vi "Magna Power Constants.vi"() -> ()   [LabVIEW 2012]
panel:
  out "Field Calibration":T1={"Fluke Voltages"=[-0.898, -0.907, -0.921, -0.93, -0.94, -0.952, -0.964, -0.976, -0.988, -1.0, -1.012, -1.025, -1.037, -1.05, -1.062, -1.074, -1.086, -1.099, -1.111, -1.123, -1.135, -1.149, -1.161, -1.174, -1.186, -1.191, -1.197, -1.203, -1.208, -1.214, -1.22, -1.225, -1.23, -1.236, -1.241, -1.246, -1.251, -1.257, -1.263, -1.269, -1.275, -1.28, -1.285, -1.29, -1.295, -1.3, -1.305, -1.309, -1.313, -1.318, -1.322, -1.326, -1.33, -1.334, -1.337, -1.341, -1.344, -1.348, -1.351, -1.354, -1.358, -1.361, -1.364, -1.366, -1.369, -1.372, -1.3748, -1.3775, -1.38, -1.3825, -1.3849, -1.3875, -1.3897, -1.3921, -1.3942, -1.3965, -1.3996, -1.4026, -1.4055, -1.4082, -1.4109, -1.4134, -1.4159, -1.4184, -1.4205, -1.4229, -1.425, -1.4272, -1.4293, -1.4314, -1.4331, -0.9047, -0.9062, -0.913, -0.9163, -0.9235, -0.9271, -0.9341, -0.89598, -0.89247, -0.88898, -0.88568, -0.88203, -0.87833, -0.87495, -0.87474, -0.87134, -0.86785, -0.86466, -0.86127, -0.85792, -0.85453, -0.85123, -0.84792, -0.83742, -0.82773, -0.81808, -0.80865, -0.79937, -0.79043, -0.78145, -0.77261, -0.76419, -0.75595, -0.74795, -0.73984, -0.73183, -0.72447, -0.71682, -0.70957, -0.70236, -0.69555, -0.68879, -0.68235, -0.67601, -0.67006, -0.66447, -0.65904, -0.65409, -0.64949, -0.64665, -0.64399, -0.6411, -0.62648, -0.62463, -0.63583, -0.63404, -0.63113, -0.62861, -0.62767, -0.62314, -0.6205, -0.61798, -0.61351, -0.61151, -0.60949, -0.60732, -0.60535, -0.60349, -0.60167, -0.59983, -0.59814, -0.59651, -0.59498, -0.59348, -0.59204, -0.59063, -0.58928, -0.58803, -0.5868, -0.58563, -0.58455, -0.58349, -0.58248, -0.58145, -0.58051, -0.57962, -0.57872, -0.57781, -0.57701, -0.57621, -0.57545, -0.57468, -0.57434], "Field Values"=[0.00828, 0.0338, 0.0696, 0.1011, 0.1325, 0.1653, 0.1983, 0.2308, 0.2632, 0.297, 0.329, 0.362, 0.394, 0.427, 0.459, 0.489, 0.521, 0.552, 0.584, 0.613, 0.645, 0.678, 0.708, 0.737, 0.767, 0.781, 0.793, 0.808, 0.821, 0.835, 0.849, 0.862, 0.874, 0.887, 0.899, 0.912, 0.923, 0.937, 0.952, 0.966, 0.979, 0.992, 1.004, 1.016, 1.028, 1.039, 1.051, 1.061, 1.072, 1.08, 1.091, 1.1, 1.109, 1.118, 1.127, 1.135, 1.144, 1.152, 1.159, 1.167, 1.175, 1.183, 1.189, 1.197, 1.205, 1.211, 1.218, 1.224, 1.231, 1.236, 1.242, 1.247, 1.253, 1.26, 1.264, 1.27, 1.276, 1.284, 1.29, 1.299, 1.305, 1.311, 1.316, 1.321, 1.327, 1.334, 1.339, 1.343, 1.35, 1.355, 1.361, 0.02542, 0.0298, 0.0499, 0.06, 0.0808, 0.0911, 0.1115, -0.002562, -0.01245, -0.0232, -0.0322, -0.0383, -0.0558, -0.0664, -0.0678, -0.0776, -0.0887, -0.0989, -0.1095, -0.1206, -0.132, -0.1428, -0.1529, -0.1875, -0.2199, -0.2512, -0.285, -0.317, -0.35, -0.38, -0.415, -0.445, -0.477, -0.507, -0.54, -0.573, -0.6, -0.632, -0.662, -0.69, -0.72, -0.749, -0.777, -0.811, -0.838, -0.858, -0.884, -0.908, -0.931, -0.946, -0.958, -0.977, -1.058, -1.068, -1.009, -1.019, -1.024, -1.039, -1.044, -1.074, -1.088, -1.104, -1.123, -1.135, -1.147, -1.159, -1.17, -1.181, -1.192, -1.202, -1.212, -1.222, -1.232, -1.241, -1.249, -1.258, -1.266, -1.274, -1.282, -1.289, -1.296, -1.303, -1.309, -1.314, -1.321, -1.326, -1.332, -1.338, -1.343, -1.348, -1.353, -1.359, -1.361]}
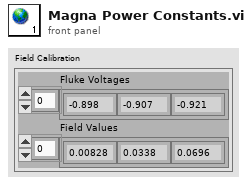
[diagram p1: front panel]
types:
  T1 = cluster{"Fluke Voltages":dbl[], "Field Values":dbl[]}
diagram:
